vi "GVmotor_EP_SP.vi"(8 "error in":errorcluster, 9 "pos":i32, 10 "wait_ms":u32=100, 11 "VISA in":refnum<visa-resource-name>) -> (0 "error out":errorcluster, 3 "VISA out":refnum<visa-resource-name>)   [LabVIEW 2019]
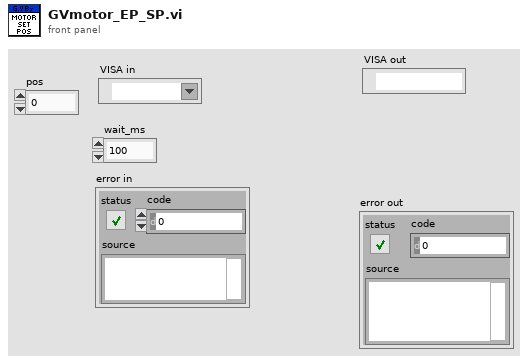
[diagram p1: front panel]
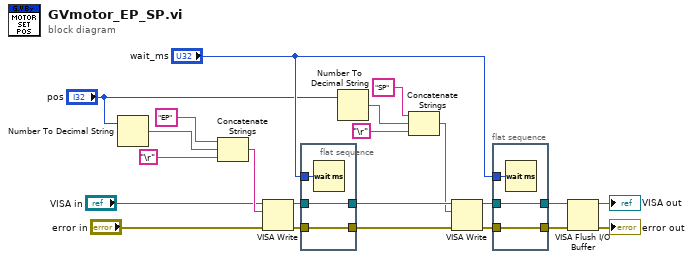
[diagram p0: block diagram]
diagram:
  n1 = Number To Decimal String(number="pos") -> (decimal integer string=w16:string)  [unwired: 1 in]
  n2 = Concatenate Strings("EP" ("string"), w16, "\r") -> (w22:string)
  n3 = VISA Write(VISA resource name="VISA in", write buffer=w22, error in (no error)="error in") -> (VISA resource name out=w18:refnum<visa-resource-name>, error out=w19:errorcluster)  [unwired: 1 out]
  n4 = flat-sequence {
    tunnel: [w25] -> w10
    tunnel: w19 -> [w25]
    tunnel: [w24] -> w11
    tunnel: w18 -> [w24]
    tunnel: "wait_ms" -> [w23]
    frame #0 {
      n5 = Wait (ms)(milliseconds to wait=w23) -> ()  [unwired: 1 out]
    }
  }
  n6 = Number To Decimal String(number="pos") -> (decimal integer string=w4:string)  [unwired: 1 in]
  n7 = Concatenate Strings("SP" ("string"), w4, "\r") -> (w2:string)
  n8 = VISA Write(VISA resource name=w11, write buffer=w2, error in (no error)=w10) -> (VISA resource name out=w9:refnum<visa-resource-name>, error out=w8:errorcluster)  [unwired: 1 out]
  n9 = flat-sequence {
    tunnel: [w28] -> w7
    tunnel: w8 -> [w28]
    tunnel: [w27] -> w12
    tunnel: w9 -> [w27]
    tunnel: [w26] -> _
    tunnel: "wait_ms" -> [w26]
    frame #0 {
      n10 = Wait (ms)(milliseconds to wait=w26) -> ()  [unwired: 1 out]
    }
  }
  n11 = VISA Flush I/O Buffer(VISA resource name=w12, error in (no error)=w7) -> (VISA resource name out=→"VISA out":refnum<visa-resource-name>, error out=→"error out":errorcluster)  [unwired: 1 in]
